vi "GlobalWhatAroundMe.vi"() -> ()   [LabVIEW 2012]
doc: "This Global Variable contains an array of ranges and bearings from robotis primary sensor suite"
panel:
  out "WhatAroundMe?":cluster{"T":dbl, "Range":dbl, "Bearing":dbl}[](array[cluster])
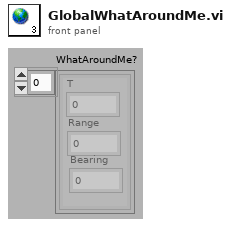
[diagram p1: front panel]
diagram:
